vi "FTW-CodeGen-DisplayName.vi"(0 "State In":T1) -> (4 "Name":string)   [LabVIEW 2015, in "FTW-Array-Shuffle.xnode"]
uses:
  FTW-Array-Shuffle.xnode
  FTW-CodeGen-State.ctl
panel:
  # "Inputs"
  # "Outputs"
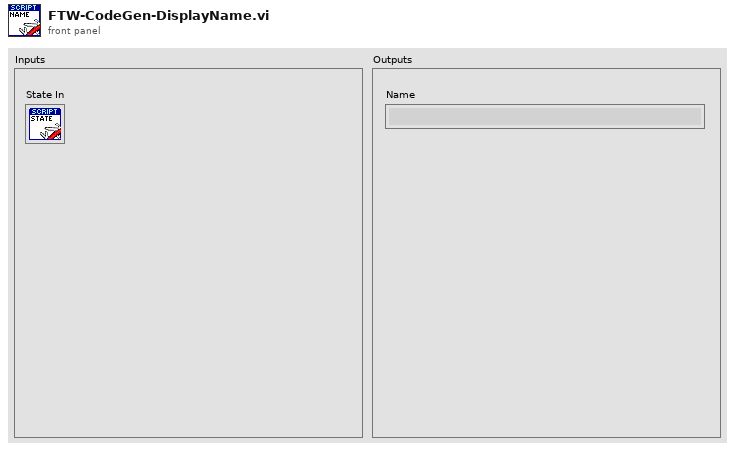
[diagram p1: front panel]
types:
  T1 = typedef "FTW-Array-Shuffle.xnode/FTW-CodeGen-State.ctl" = cluster{"Dummy":string}
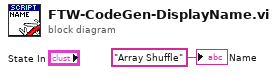
[diagram p0: block diagram]
diagram:
  "Name" <- "Array Shuffle" ("Name")
